vi "RX.vi"(7 "Timeout (10000)":i32=10000, 8 "error in (no error)":errorcluster, 9 "Transaction Notifier":refnum<notifier>, 10 "Transaction LUT in":refnum<data-value>, 11 "ADU in":refnum<class "MB_ADU_TCP.lvclass">) -> (0 "error out":errorcluster, 1 "PDU_resp":T1={"Function Code"=1, "Data"=[], "RTU_DataBytes"=0}, 2 "Transaction LUT out":refnum<data-value>, 3 "ADU out":refnum<class "MB_ADU_TCP.lvclass">)   [LabVIEW 2012, in "MB Master.lvlib" / "MB_Master_TCP.lvclass"]
uses:
  MB_Master_TCP.lvclass
  MB_ADU_TCP/MB_ADU_TCP.lvclass
  MB_PDU/MB_PDU_Cluster.ctl
  MB_ADU_TCP/MB_ADU_TCP.lvclass/MB_ADU_TCP.ctl
  MB_ADU_TCP/Read Transaction ID.vi
  MB Master.lvlib
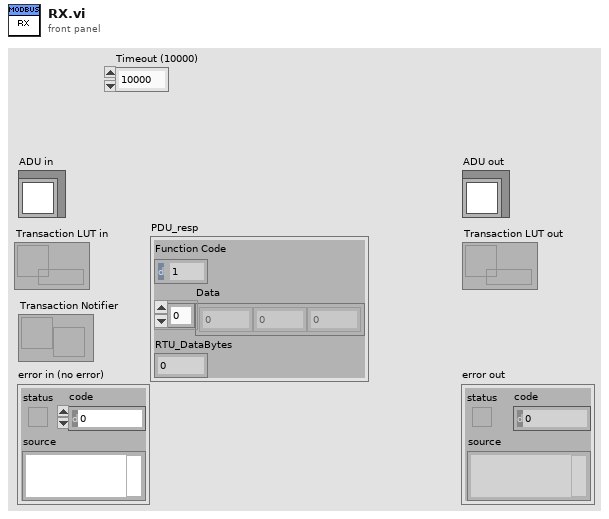
[diagram p1: front panel]
types:
  T1 = typedef "MB Master.lvlib/MB_PDU_Cluster.ctl" = cluster{"Function Code":u8, "Data":u8[], "RTU_DataBytes":i32}
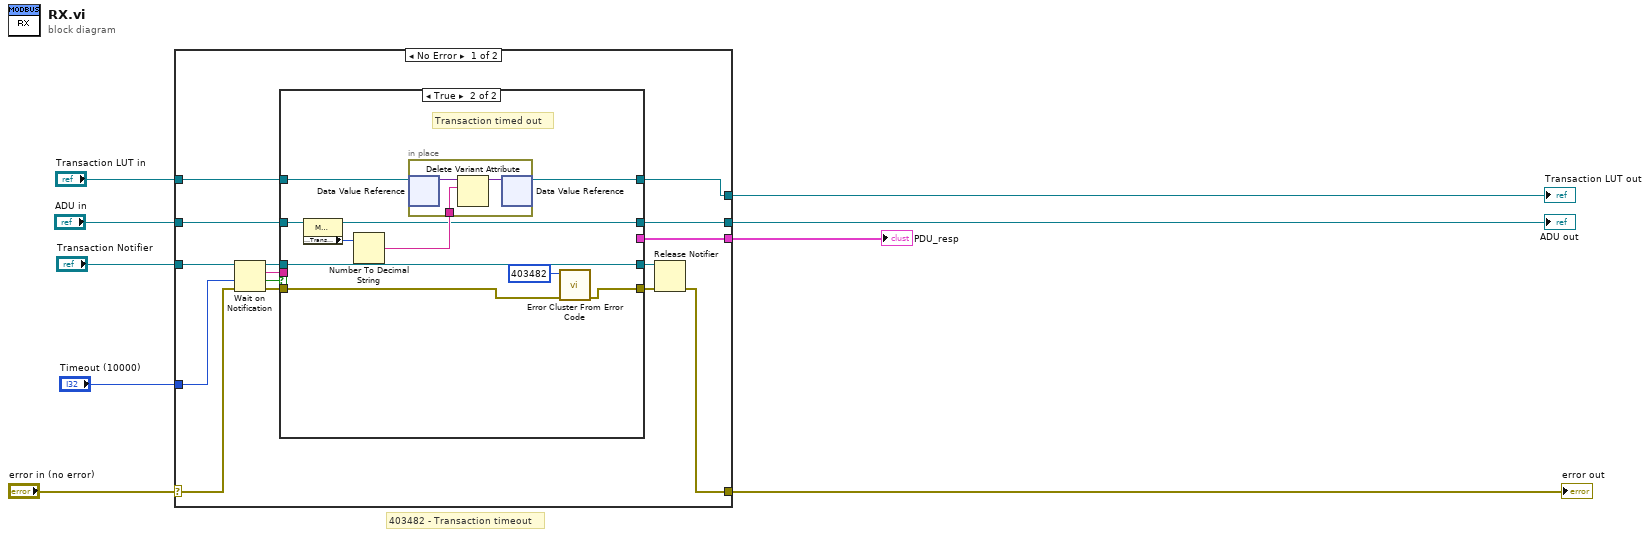
[diagram p0: block diagram]
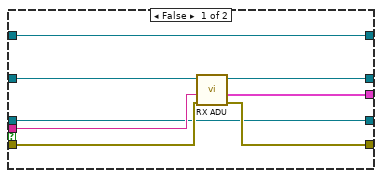
[diagram p2: hidden frame]
diagram:
  # "403482 - Transaction timeout"
  n1 = case shown="No Error" "error in (no error)" {
    selector: "error in (no error)" -> [w19 w48]
    tunnel: [w11 w48] -> w8
    tunnel: "Transaction LUT in" -> [w15 w47]
    tunnel: [w13 w47] -> w6
    tunnel: "ADU in" -> [w22 w46]
    tunnel: [w21 w46] -> w4
    tunnel: "Transaction Notifier" -> [w20 _]
    tunnel: [w18 _] -> w2
    tunnel: "Timeout (10000)" -> [w17 _]
    frame No Error {
      n2 = Wait on Notification(notifier=w20, timeout in ms (-1)=w17, error in (no error)=w19) -> (notifier out=w14:refnum<notifier>, notification=w24:string, timed out?=w16:bool, error out=w23:errorcluster)  [unwired: 1 in]
      n3 = case shown="True" w16 {
        tunnel: w24 -> [w32 _]
        tunnel: [w31 w34] -> w12
        tunnel: w23 -> [w30 w35]
        tunnel: w22 -> [w29 w41]
        tunnel: [w28 w36] -> w21
        tunnel: [w27 _] -> w18
        tunnel: w15 -> [w26 w42]
        tunnel: w14 -> [w25 w37]
        tunnel: [w26 w38] -> w13
        tunnel: [w25 w37] -> w10
        frame False {
          n4 = call "RX ADU.vi"("error in (no error)"=w30, "RX Data"=w32, "MB_ADU_TCP in"=w29) -> ("error out"=w31:errorcluster, "PDU_resp"=w27:T1, "MB_ADU_TCP out"=w28:refnum<class "MB_ADU_TCP.lvclass">)  [unwired: 6 in]
        }
        frame True {
          # "Transaction timed out"
          n5 = property class="MB_ADU_TCP"(reference=w41) -> (reference out=w36:refnum<class "MB_ADU_TCP.lvclass">, "Properties:Transaction ID"=w40:u16)  [unwired: 1 in, 1 out]
          n6 = Number To Decimal String(number=w40) -> (decimal integer string=w39:string)  [unwired: 1 in]
          n7 = in-place {
            in-place-border: w39 -> [w44]
            n8 = in-place-dvr #1(w42) -> (w43:variant)  [unwired: 1 out]
            n9 = Delete Variant Attribute(6:w44, 7:w43) -> (3:w45:variant)  [unwired: 1 in, 2 out]
            n10 = in-place-dvr #1(w45) -> (w38:refnum<data-value>)  [unwired: 1 out]
          }
          n11 = call <vilib>:"Error Cluster From Error Code.vi"("error in (no error)"=w35, "error code (0)"=403482) -> ("error out"=w34:errorcluster)  [unwired: 7 in]
        }
      }
      n12 = Release Notifier(notifier=w10, error in (no error)=w12) -> (error out=w11:errorcluster)  [unwired: 1 in, 2 out]
    }
    frame Error {
    }
  }
  "error out" <- w8
  "Transaction LUT out" <- w6
  "ADU out" <- w4
  "PDU_resp" <- w2
